vi "perfer given heading.vi"(9 "desired heading":i8, 10 "min obstacle dist":u16, 11 "driveable path lengths":u16[](array[numeric])=[128, 128, 128, 128, 128, 128, 128, 128, 128, 128, 128, 128, 128, 128, 128, 128]) -> (0 "driveable paths?":bool, 3 "wheel angle":i8)   [LabVIEW 2010]
panel:
  in  "possible wheel angles":i8[](array[numeric])=[-35, -30, -25, -20, -15, -10, -5, -1, 1, 5, 10, 15, 20, 25, 30, 35]
  out "Heartbeat":bool
  out "coerced x":i8
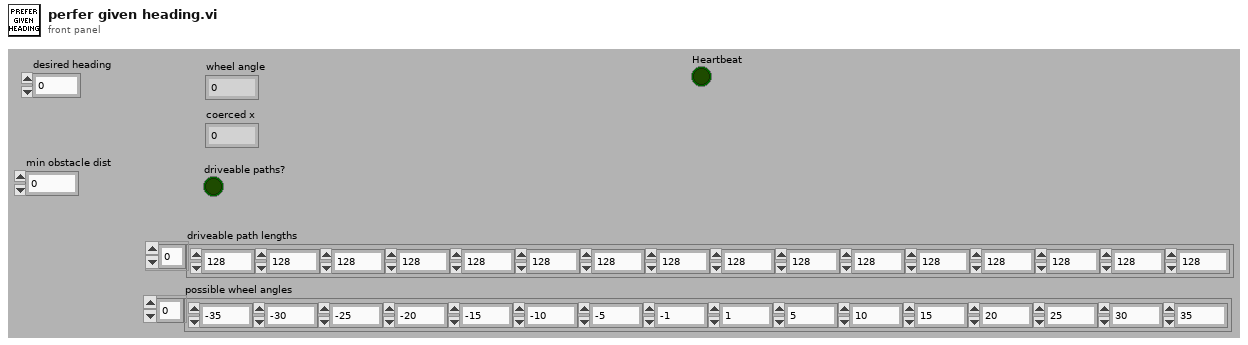
[diagram p1: front panel]
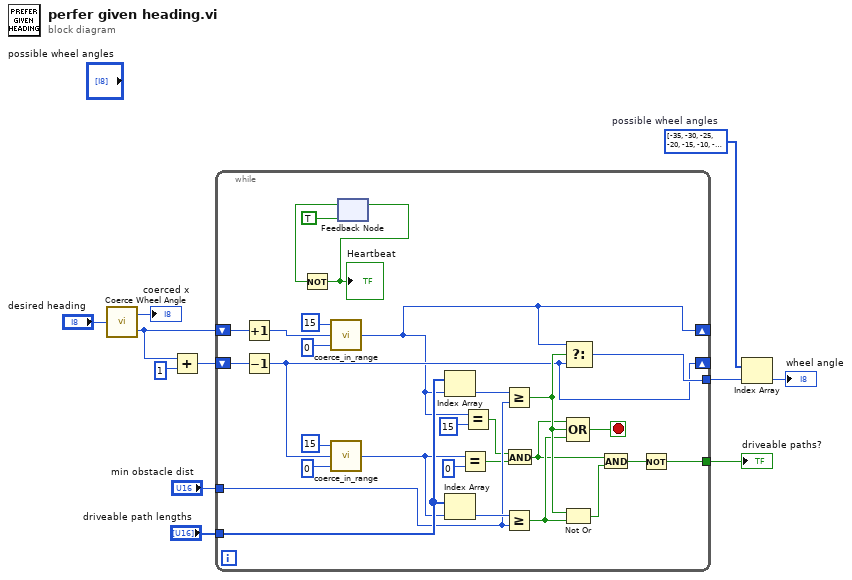
[diagram p0: block diagram]
diagram:
  w8 = i8[] [-35, -30, -25, -20, -15, -10, -5, -1, 1, 5, 10, 15, 20, 25, 30, 35]  # possible wheel angles
  n1 = call "Coerce Wheel Angle.vi"("Angle In"="desired heading") -> ("Wheel Angle"=→"coerced x":i8, "Path Index"=w1:i32)
  n2 = Add(x=w1, y=i8 1) -> (x+y=w2:i32)
  n3 = while {
    tunnel: "driveable path lengths" -> [w40]
    tunnel: "min obstacle dist" -> [w37]
    tunnel: [w34] -> w10
    shift-right: [w12] -> _
    shift-left: w1 -> [w30]
    shift-right: [w22] -> _
    shift-left: w2 -> [w29]
    tunnel: [w28] -> w9
    stop <- w35 stop-if-true
    n4 = Increment(x=w30) -> (x+1=w27:i32)
    n5 = Decrement(x=w29) -> (x-1=w22:i32)
    n6 = call "coerce_in_range.vi"("min"=i8 0, "x"=w27, "max"=i8 15) -> ("coerced x"=w12:i8)  [unwired: 2 in]
    n7 = call "coerce_in_range.vi"("min"=i8 0, "x"=w22, "max"=i8 15) -> ("coerced x"=w18:i8)  [unwired: 2 in]
    n8 = feedback #1(TRUE) -> (w14:bool)
    n9 = Not(x=w14) -> (.not. x?=w15:bool)
    "Heartbeat" <- w15
    n10 = feedback-in #1(w15) -> ()
    n11 = Index Array(array=w40, index=w12) -> (element=w38:u16)
    n12 = Index Array(array=w40, index=w18) -> (element=w39:u16)
    n13 = Equal?(x=w18, y=0) -> (x = y?=w17:bool)
    n14 = Equal?(x=w12, y=15) -> (x = y?=w21:bool)
    n15 = Greater Or Equal?(x=w38, y=w37) -> (x >= y?=w33:bool)
    n16 = Greater Or Equal?(x=w39, y=w37) -> (x >= y?=w32:bool)
    n17 = And(x=w21, y=w17) -> (x .and. y?=w16:bool)
    n18 = Not Or(1:w32, 2:w33) -> (0:w31:bool)
    n19 = Select(t=w12, s=w33, f=w22) -> (s? t:f=w28:i32)
    n20 = Compound Arithmetic op=OR(w16, w33, w32) -> (w35:bool)
    n21 = And(x=w16, y=w31) -> (x .and. y?=w20:bool)
    n22 = Not(x=w20) -> (.not. x?=w34:bool)
  }
  "driveable paths?" <- w10
  n23 = Index Array(array=w8, index=w9) -> (element=→"wheel angle":i8)
